vi "CliEBRead.vi"(0 "ref in":u64, 1 "DB Number":i32=1, 5 "Start":i32, 7 "Amount":i32, 9 "data in":string, 11 "error in (no error)":errorcluster, 12 "Word Length":i32(ring)=2 items=["Bit"=1, "Byte"=2, "Word"=4, "DWord"=6, "Real"=8, "Counter"=28, "Timer"=29]) -> (4 "ref out":u64, 6 "Result":i32, 10 "data out":string, 15 "error out":errorcluster)   [LabVIEW 2010, in "Snap7.lvlib"]
uses:
  Snap7.lvlib
  windows/lv_snap7.dll
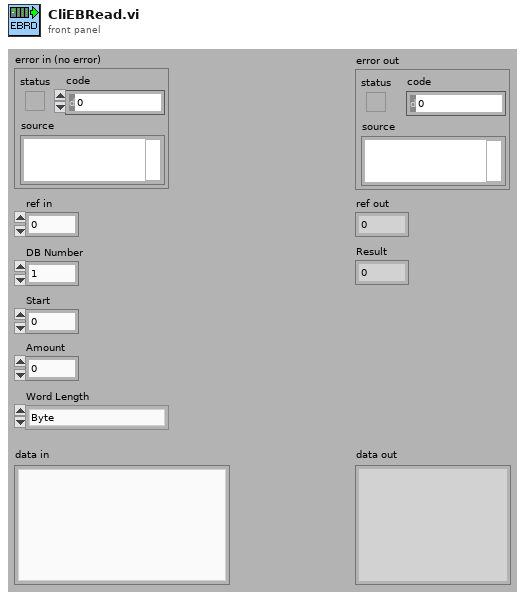
[diagram p1: front panel]
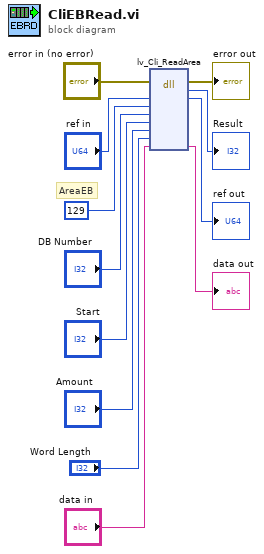
[diagram p0: block diagram]
diagram:
  # "AreaEB"
  n1 = dll-call lib="C:/snap7-src-1.0.0/LabVIEW/lib/windows/lv_snap7.dll" fn="lv_Cli_ReadArea"(error in="error in (no error)", "Client"="ref in", "Area"=129, "DBNumber"="DB Number", "Start"="Start", "Amount"="Amount", "WordLen"="Word Length", "pUsrData"="data in") -> (error out=→"error out":errorcluster, "return type"=→"Result":i32, "Client"=→"ref out":u64, "pUsrData"=→"data out":string)  [unwired: 7 in, 1 out]
